vi "STP_Client.vi"() -> ()   [LabVIEW 2016]
uses:
  <vilib>/NI/STM/SubVIs/MetaDataElement.ctl
  Typedefs/Remote-SMO-Commands-Enum.ctl
  <vilib>/NI/STM/TCP/TCP Read Options.ctl
  <vilib>/NI/STM/TCP/Read Meta Data (TCP Ref).vi
  <vilib>/NI/STM/TCP/Get Connection Reference (TCP).vi
  <vilib>/NI/STM/TCP/Read Meta Data (TCP Clst).vi
  <vilib>/NI/STM/TCP/Write Message (TCP).vi
  <vilib>/NI/STM/TCP/Read Message (TCP).vi
  <userlib>/_OpenG.lib/error/error.llb/Filter Error Codes (Array)__ogtk.vi
  <vilib>/NI/STM/NI STM.lvlib
  RemoteControl.lvclass
panel:
  in  "stop":bool
  out "since last call ms":u32
  out "x+1":dbl
  out "duration ms":u32
  in  "address":string
  out "available commands = enum?":bool
  in  "Enum":T1
  out "meta data (available commands)":T2[](array[typedef])
  out "data received from server":string
  in  "data to send":string
  out "error out":errorcluster
  # "CLIENT (API)"
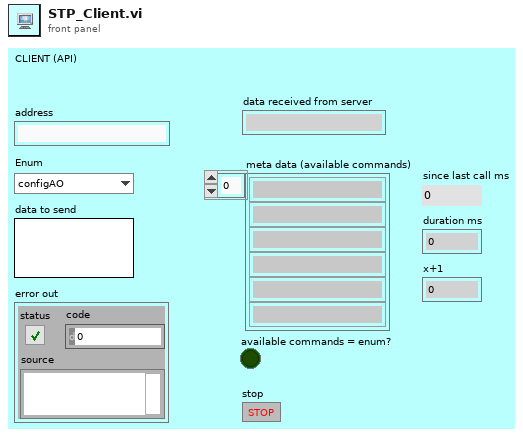
[diagram p1: front panel]
types:
  T1 = typedef "RemoteControl.lvclass/Remote-SMO-Commands-Enum.ctl" = enum16{"configAO", "configLockin", "ACK", "CLOSE"}
  T2 = typedef "NI STM.lvlib/MetaDataElement.ctl" = string
  T3 = typedef "NI STM.lvlib/TCP Read Options.ctl" = cluster{"ignore timeout error":bool, "timeout ms (1000)":i32}
  T4 = typedef "NI STM.lvlib/TCP Connection Info.ctl" = cluster{"connection ID":refnum<k5>, "meta data":T2[]}
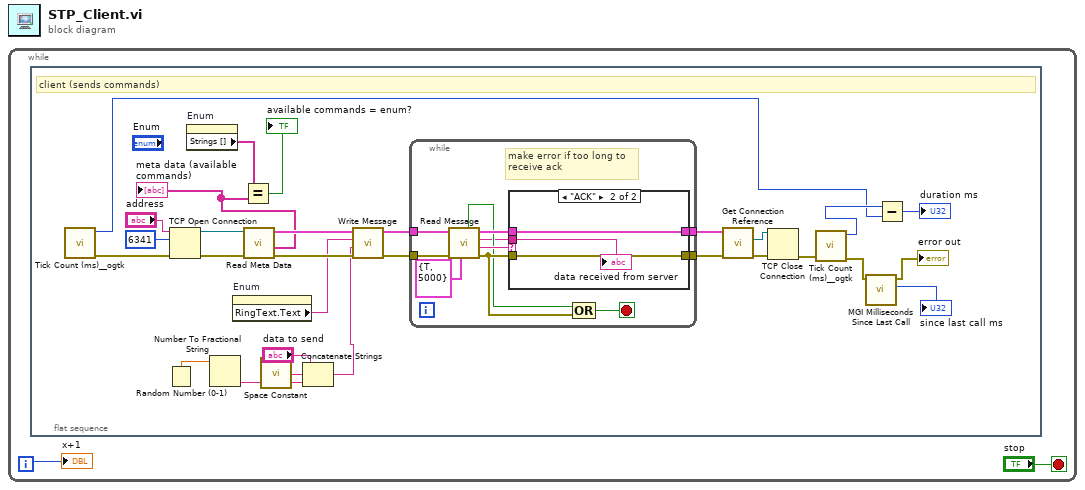
[diagram p0: block diagram]
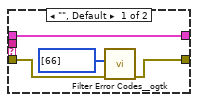
[diagram p2: hidden frame]
diagram:
  n1 = while {
    i -> [w1]
    stop <- "stop" stop-if-true
    n2 = flat-sequence {
      frame #0 {
        # "client (sends commands)"
        n3 = call <userlib>:"Tick Count (ms)__ogtk.vi"() -> ("error out"=w18:errorcluster, "millisecond timer value"=w11:u32)  [unwired: 10 in]
        n4 = Random Number (0-1)() -> (number: 0 to 1=w6:dbl)
        n5 = TCP Open Connection(address="address", remote port or service name=u16 6341, error in (no error)=w18) -> (connection ID=w26:refnum<k5>, error out=w27:errorcluster)  [unwired: 2 in]
        n6 = property on="Enum" class="Enum (strict)"() -> ("Strings []"=w25:string[])  [unwired: 2 in, 2 out]
        n7 = Number To Fractional String(number=w6) -> (F-format string=w10:string)  [unwired: 3 in]
        n8 = property on="Enum" class="Enum (strict)"() -> ("RingText.Text"=w17:string)  [unwired: 2 in, 2 out]
        n9 = call-poly <vilib>:"Read Meta Data.vi"("error in"=w27, "connection ID"=w26) -> ("error out"=w30:errorcluster, "meta data"=w22:T2[], "connection info out"=w31:T4)  [unwired: 7 in]
        "meta data (available commands)" <- w22
        n10 = Equal?(x=w25, y=w22) -> (x = y?=→"available commands = enum?":bool)
        n11 = call <vilib>:"Space Constant.vi"() -> ("String"=w7:string)
        n12 = Concatenate Strings("data to send", w7, w10) -> (w9:string)
        n13 = call-poly <vilib>:"Write Message.vi"("error in"=w30, "data"=w9, "name"=w17, "connection info in"=w31) -> ("error out"=w29:errorcluster, "connection info out"=w28:T4)  [unwired: 6 in]
        n14 = while {
          tunnel: w29 -> [w42]
          tunnel: w28 -> [w41]
          tunnel: [w39] -> w16
          tunnel: [w37] -> w15
          stop <- w36 stop-if-true
          # "make error if too long to\nreceive ack"
          n15 = call-poly <vilib>:"Read Message.vi"("options"=T3 {"ignore timeout error"=TRUE, "timeout ms (1000)"=5000}, "error in"=w42, "connection info in"=w41) -> ("error out"=w35:errorcluster, "name"=w40:T2, "data string"=w33:string, "connection info out"=w38:T4, "timed out?"=w34:bool)  [unwired: 1 in, 3 out]
          n16 = case shown="\"ACK\"" w40 {
            tunnel: w35 -> [w43 w49]
            tunnel: [w45 w49] -> w39
            tunnel: w38 -> [w46 w48]
            tunnel: [w46 w48] -> w37
            tunnel: w33 -> [_ w47]
            frame "", Default {
              n17 = call-poly <userlib>:"Filter Error Codes__ogtk.vi"("Error In"=w43, "Error Codes to Filter"=i32[] [66]) -> ("Error Out"=w45:errorcluster)  [unwired: 7 in, 2 out]
            }
            frame "ACK" {
              "data received from server" <- w47
            }
          }
          n18 = Compound Arithmetic op=OR(w34, w35) -> (w36:bool)
        }
        n19 = call-poly <vilib>:"Get Connection Reference.vi"("error in"=w16, "connection info in"=w15) -> ("error out"=w20:errorcluster, "connection ID out"=w19:refnum<k5>)  [unwired: 7 in, 1 out]
        n20 = TCP Close Connection(connection ID=w19, error in (no error)=w20) -> (error out=w14:errorcluster)  [unwired: 1 in, 1 out]
        n21 = call <userlib>:"Tick Count (ms)__ogtk.vi"("error in (no error)"=w14) -> ("error out"=w5:errorcluster, "millisecond timer value"=w12:u32)  [unwired: 9 in]
        n22 = call <userlib>:"MGI Milliseconds Since Last Call.vi"("Error In"=w5) -> ("ms"=→"since last call ms":u32, "Error Out"=→"error out":errorcluster)  [unwired: 5 in]
        n23 = Subtract(x=w12, y=w11) -> (x-y=→"duration ms":u32)
      }
    }
    "x+1" <- w1
  }
